vi "Read File.vi"(7 "Section":string, 8 "error in (no error)":errorcluster, 10 "Parameters in":refnum<class "Parameter.lvclass">[](array[class]), 11 "Parameter Generic File in":refnum<class "Parameter Generic File.lvclass">) -> (0 "error out":errorcluster, 2 "Parameters out":refnum<class "Parameter.lvclass">[](array[class]), 3 "Parameter Generic File out":refnum<class "Parameter Generic File.lvclass">)   [LabVIEW 2016, in "CD Parameter Manager API.lvlib" / "Parameter Generic File.lvclass"]
uses:
  Parameter Generic File.lvclass
  Parameter Class/Parameter.lvclass
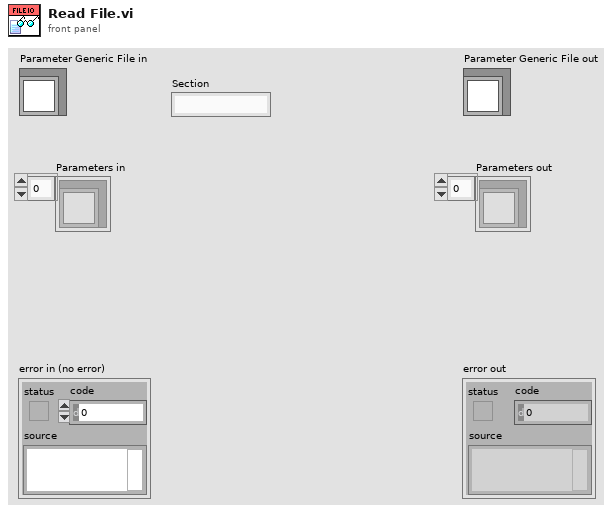
[diagram p1: front panel]
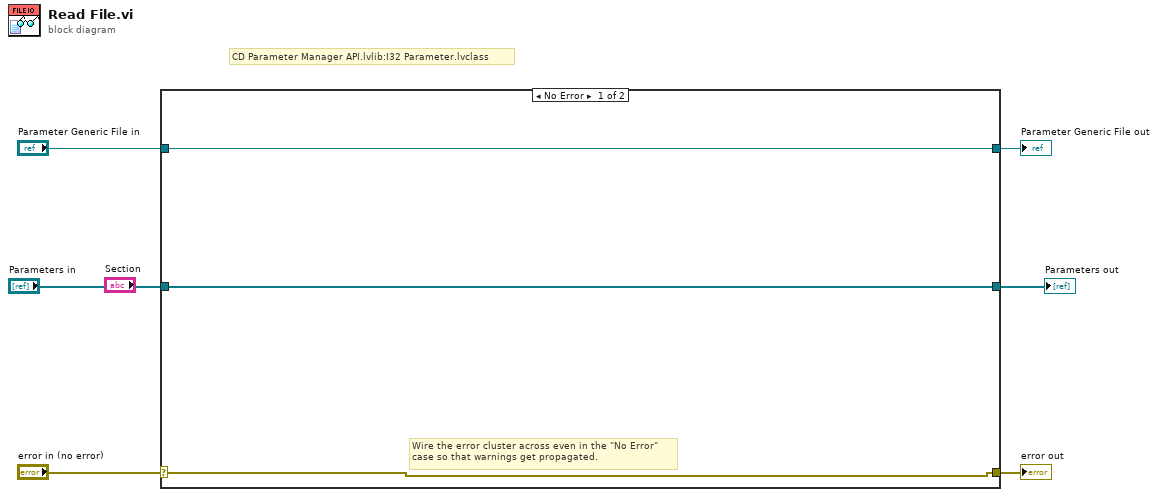
[diagram p0: block diagram]
diagram:
  # "CD Parameter Manager API.lvlib:I32 Parameter.lvclass"
  n1 = case shown="No Error" "error in (no error)" {
    selector: "error in (no error)" -> [w8 w12]
    tunnel: [w8 w12] -> w5
    tunnel: [w9 w11] -> w3
    tunnel: "Parameter Generic File in" -> [w9 w11]
    tunnel: [w7 w10] -> w1
    tunnel: "Parameters in" -> [w7 w10]
    frame No Error {
      # "Wire the error cluster across even in the \"No Error\"\ncase so that warnings get propagated."
    }
    frame Error {
    }
  }
  "error out" <- w5
  "Parameter Generic File out" <- w3
  "Parameters out" <- w1
